vi "Pressure.vi"(8 "error in (no error)":errorcluster, 10 "Pressure":i16, 11 "Ultimus V in":refnum<class "Ultimus V.lvclass">) -> (0 "error out":errorcluster, 3 "Ultimus V out":refnum<class "Ultimus V.lvclass">)   [LabVIEW 2020, in "Ultimus V.lvclass"]
uses:
  Ultimus V.lvclass
  Ultimus V.lvclass/Ultimus V.ctl
  <instrlib>/Agilent 34401/Agilent 34401.lvlib
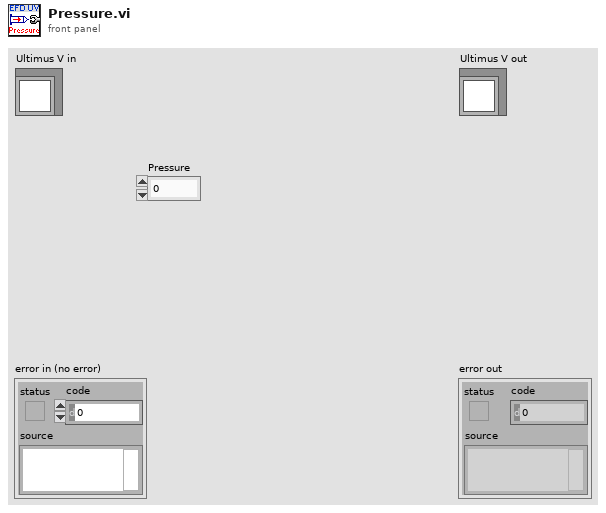
[diagram p1: front panel]
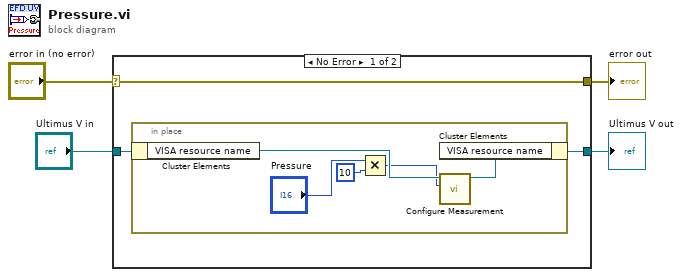
[diagram p0: block diagram]
diagram:
  n1 = case shown="No Error" "error in (no error)" {
    selector: "error in (no error)" -> [w5 w14]
    tunnel: "Ultimus V in" -> [w7 w13]
    tunnel: [w6 w13] -> w3
    tunnel: [w5 w14] -> w1
    frame No Error {
      n2 = in-place {
        n3 = in-place-cluster #1(w7) -> ("VISA resource name"=w10:refnum<visa-resource-name>)
        n4 = Multiply(x="Pressure", y=i16 10) -> (x*y=w9:i16)
        n5 = call <instrlib>:"Configure Measurement.vi"("Function (0: DC Voltage)"=w9, "VISA resource name"=w10) -> ("VISA resource name out"=w8:refnum<visa-resource-name>)  [unwired: 8 in, 1 out]
        n6 = in-place-cluster #1("VISA resource name"=w8) -> (w6:refnum<class "Ultimus V.lvclass">)
      }
    }
    frame Error {
    }
  }
  "error out" <- w1
  "Ultimus V out" <- w3
